vi "Script Add Input to Bundler.vi"(8 "error in":errorcluster, 11 "Bundler in":refnum<vi>) -> (0 "error out":errorcluster, 2 "New Input":refnum<vi>, 3 "Bundler out":refnum<vi>)   [LabVIEW 2018, in "Scripting.lvlib"]
uses:
  Scripting.lvlib
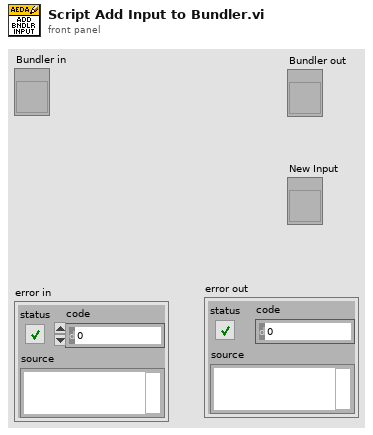
[diagram p1: front panel]
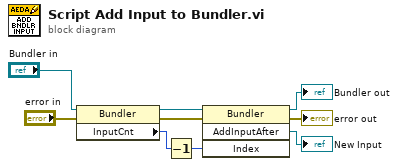
[diagram p0: block diagram]
diagram:
  n1 = property class="Bundler"(reference="Bundler in", error in="error in") -> (reference out=w7:refnum<vi>, error out=w6:errorcluster, "InputCnt"=w5:i32)
  n2 = Decrement(x=w5) -> (x-1=w1:i32)
  n3 = invoke class="Bundler" method="AddInputAfter"(reference=w7, error in=w6, "Index"=w1) -> (reference out=→"Bundler out":refnum<vi>, error out=→"error out":errorcluster, "AddInputAfter"=→"New Input":refnum<vi>)  [unwired: 1 in, 1 out]
